vi "prompts list.vi"(8 "error in":errorcluster, 10 "id":i32, 11 "message json":string) -> (0 "error out":errorcluster, 3 "response":string)   [LabVIEW 2025, in "MCP Server.lvlib"]
uses:
  MCP Server.lvlib
  97a80f9a-628e-4717-95e0-87c27c4c3e74.vi
  <vilib>/JDP Science/JSONtext/Variant to JSON Text.vi
  <vilib>/JDP Science/JSONtext/support/Format JSON Object.vi
  <vilib>/JDP Science/JSONtext/LVClass Serializer/JSONtext LVClass Serializer.lvclass
  <vilib>/JDP Science/JSONtext/JSONtext.lvlib
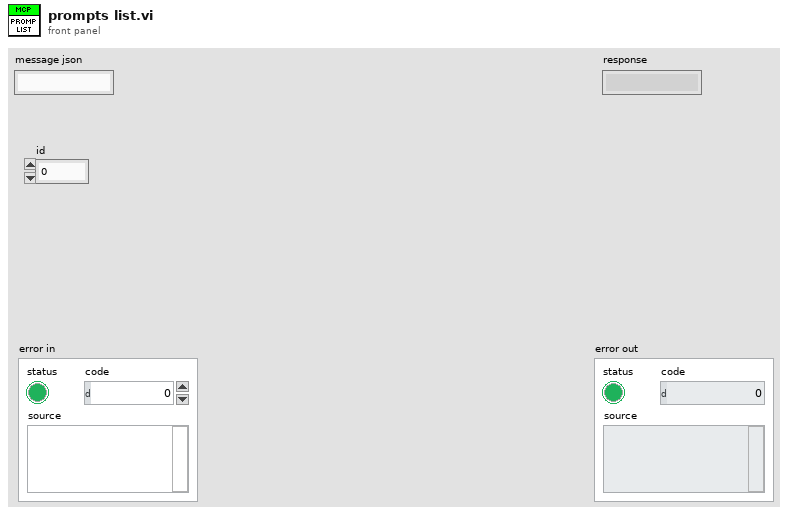
[diagram p1: front panel]
types:
  T1 = typedef "MCP Server.lvlib/Prompt Data.ctl" = cluster{"name":string, "description":string, "arguments":T2[], "return terminal name":string, "results description":string, "VI Refnum":refnum<vi>}
  T2 = typedef "MCP Server.lvlib/Prompt Argument.ctl" = cluster{"name":string, "description":string, "required":bool, "raw_name":string}
  T3 = cluster{"name":string, "description":string, "arguments":cluster{"name":string, "description":string}[]}
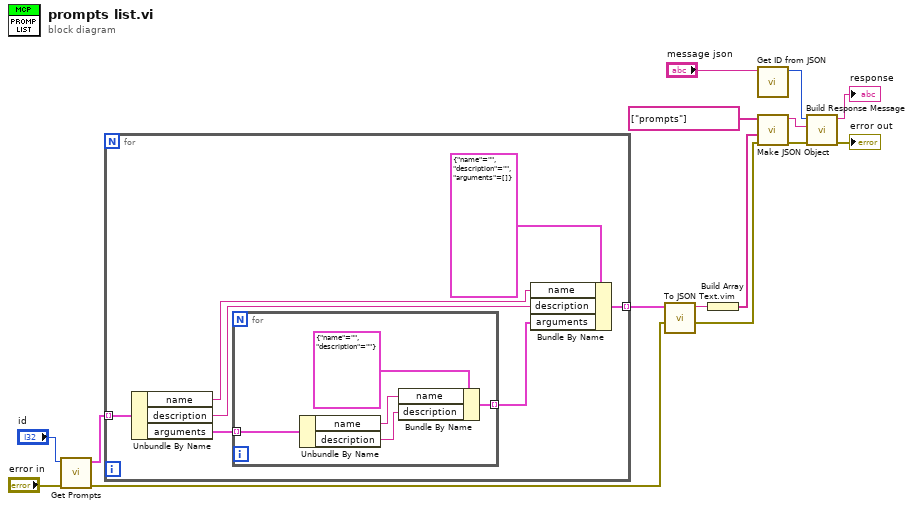
[diagram p0: block diagram]
diagram:
  n1 = call "Get Prompts.vi"("error in (no error)"="error in", "id"="id") -> ("error out"=w12:errorcluster, "Prompts"=w6:T1[])  [unwired: 8 in]
  n2 = for {
    tunnel: w6 -> [w22] mode=indexing
    tunnel: [w16] -> w5 mode=indexing
    n3 = Unbundle By Name(w22) -> ("name"=w17:string, "description"=w18:string, "arguments"=w21:T2[])
    n4 = for {
      tunnel: w21 -> [w27] mode=indexing
      tunnel: [w23] -> w19 mode=indexing
      n5 = Unbundle By Name(w27) -> ("name"=w25:string, "description"=w24:string)
      n6 = Bundle By Name(cluster=cluster{"name":string, "description":string} {"name"="", "description"=""}, "name"=w25, "description"=w24) -> (w23:cluster{"name":string, "description":string})
    }
    n7 = Bundle By Name(cluster=T3 {"name"="", "description"="", "arguments"=[]}, "name"=w17, "description"=w18, "arguments"=w19) -> (w16:T3)
  }
  n8 = call "To JSON Text.vim"("error in (no error)"=w12, "Anything"=w5) -> ("error out"=w8:errorcluster, "<JSON>"=w9:string)  [unwired: 8 in]
  n9 = Build Array(w9) -> (w10:string[])
  n10 = call "Get ID from JSON.vi"("message json"="message json") -> ("Data out"=w2:i32)  [unwired: 10 in]
  n11 = call <vilib>:"Make JSON Object.vi"("error in (no error)"=w8, "JSON Items"=w10, "Item Names"=string[] ["prompts"]) -> ("error out"=w7:errorcluster, "<JSON>"=w1:string)  [unwired: 7 in]
  n12 = call "Build Response Message.vi"("error in (no error)"=w7, "Result content"=w1, "message id in"=w2) -> ("error out"=→"error out":errorcluster, "MCP message out"=→"response":string)  [unwired: 7 in]
